vi "Argo_Drive.vi"(0 "Speed_Main":dbl=-0.047244094488188976, 1 "Turning_Still_Multiplier":dbl=1.5, 2 "Argo Drive Joystick Map":T1, 3 "Backwards_Turning_Flip":bool, 4 "Turning_PID_Enable":bool, 5 "PID Gains":T3, 6 "Turning_Main":dbl=-0.007874015748031496, 7 "Auto_Enable":bool, 8 "High_Gear":bool, 9 "Quick_Turn":bool=TRUE, 10 "Turning_Setpoint":dbl, 11 "dt (s)":dbl=10.0 format="%.3f", 14 "Yaw":dbl=654.9580428601698) -> (12 "Left_Motor":dbl format="%.2f", 13 "Right_Motor":dbl format="%.2f")   [LabVIEW 2017, in "ArgosLib.lvlib"]
uses:
  ArgosLib.lvlib
  Miscellaneous/TypeDefs/ArgoDriveJoystickMap.ctl
  Miscellaneous/TypeDefs/LookUpTableParameters.ctl
panel:
  out "Waveform Chart":cluster{"Left_Motor_Sat":dbl, "Output":dbl}(graph)
  in  "Ramp_Rate":dbl=0.2
  out "XY Turning":cluster{"Turning X ":dbl[], "Turning Y":dbl[]}(graph)={"Turning X "=[-1.0, -0.75, -0.2, -0.19, 0.0, 0.19, 0.2, 0.75, 1.0], "Turning Y"=[-1.0, -0.4, -0.1, 0.0, 0.0, 0.0, 0.1, 0.4, 1.0]}
  out "XY Speed":cluster{"Speed X":dbl[], "Speed Y":dbl[]}(graph)={"Speed X"=[-1.0, -0.75, -0.21, -0.2, 0.0, 0.2, 0.21, 0.75, 1.0], "Speed Y"=[-1.0, -0.4, -0.15, 0.0, 0.0, 0.0, 0.15, 0.4, 1.0]}
  in  "Turning Scale":dbl=1.5
  out "Delta":dbl format="%.2f"
  # "Chessy Drive"
  # "This subystem takes turning and speed controls from a xbox joystick \nand creats left and right motor values"
  # "Tunning"
  # "Inputs"
  # "Test Points"
  # "Ouputs"
  # "Joystick Map (Lookup Table)"
  # "Turning Power Mode"
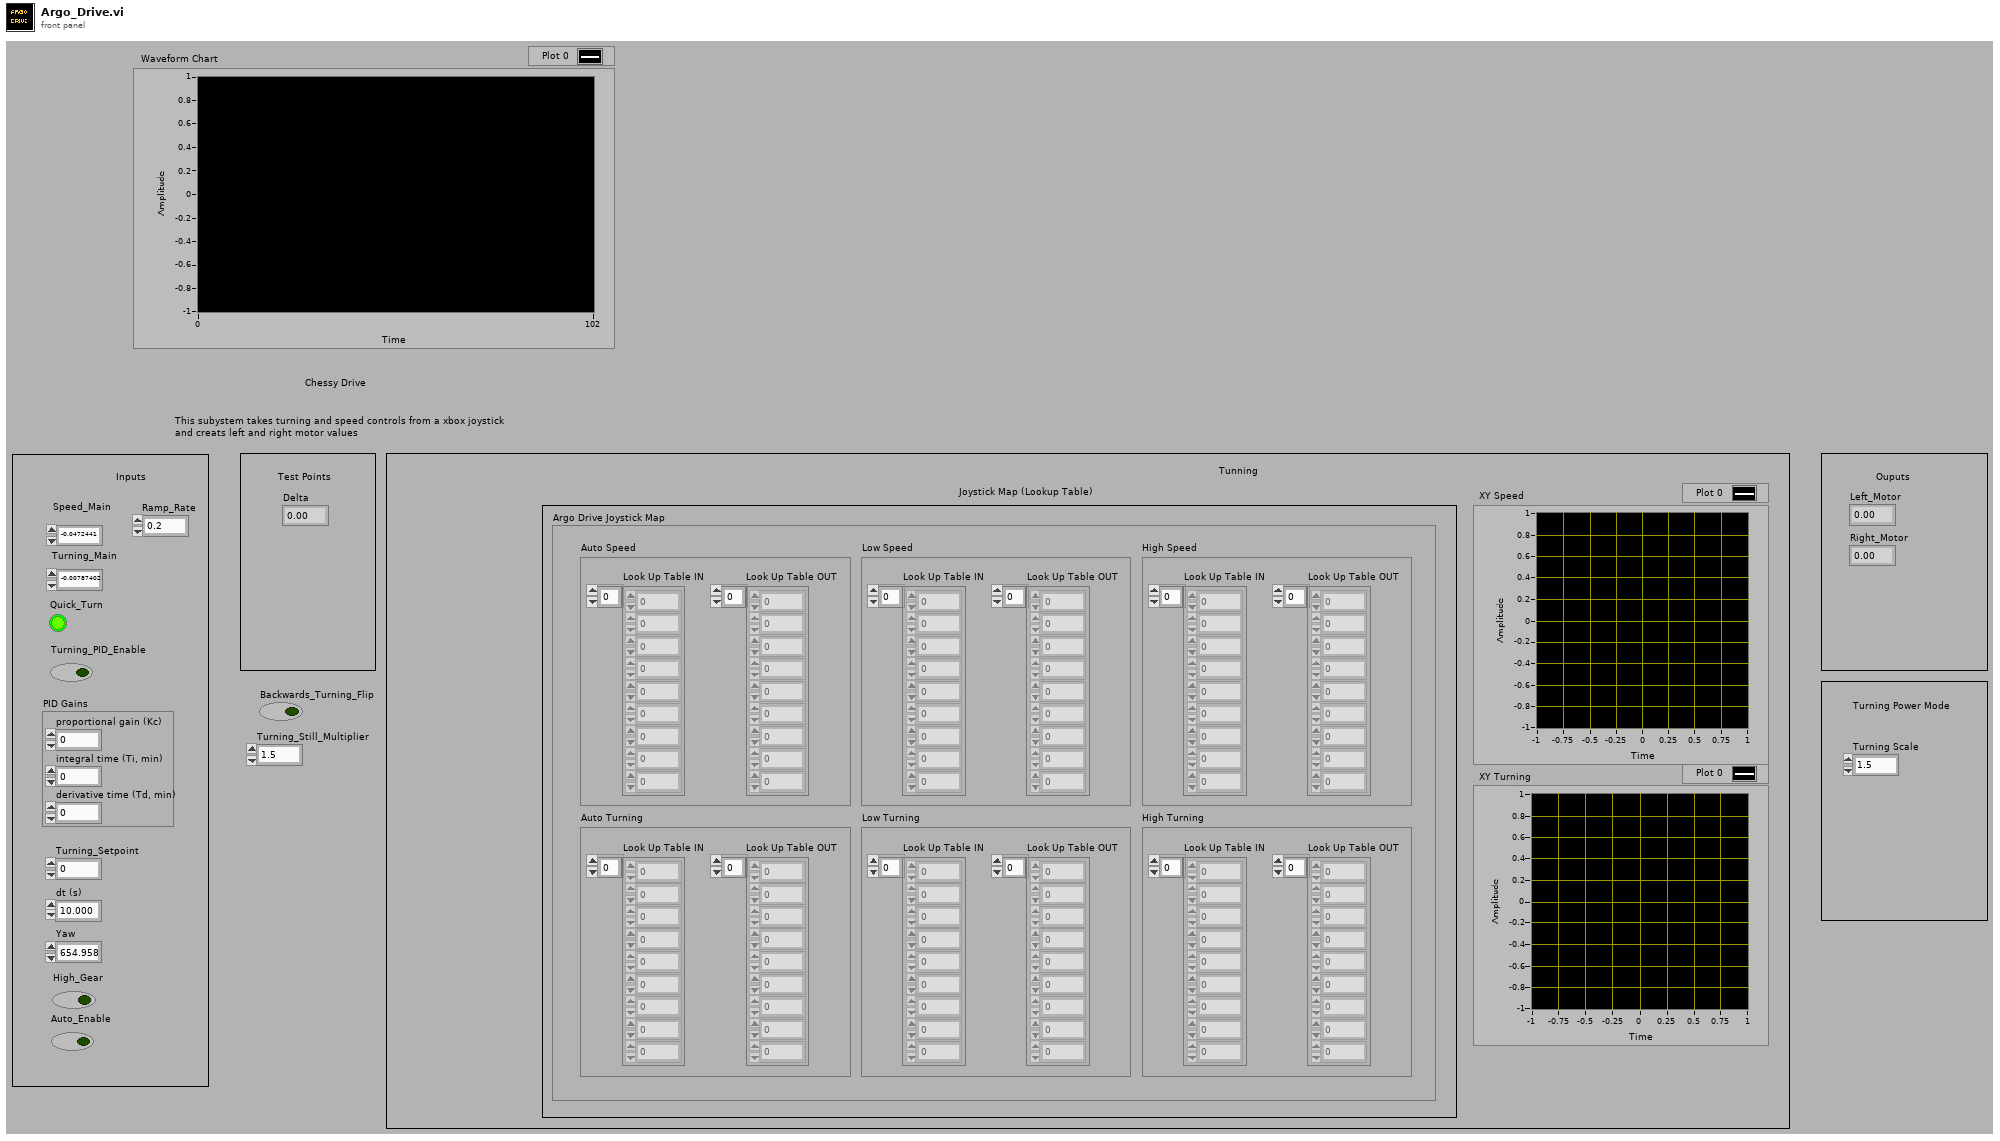
[diagram p1: front panel]
types:
  T1 = typedef "ArgosLib.lvlib/ArgoDriveJoystickMap.ctl" = cluster{"Auto Speed":T2, "Low Speed":T2, "Auto Turning":T2, "Low Turning":T2, "High Speed":T2, "High Turning":T2}
  T2 = typedef "ArgosLib.lvlib/LookUpTableParameters.ctl" = cluster{"Look Up Table OUT":dbl[], "Look Up Table IN":dbl[]}
  T3 = cluster{"proportional gain (Kc)":dbl, "integral time (Ti, min)":dbl, "derivative time (Td, min)":dbl}
  T4 = cluster{"Look Up Table IN":dbl[], "Look Up Table OUT":dbl[]}
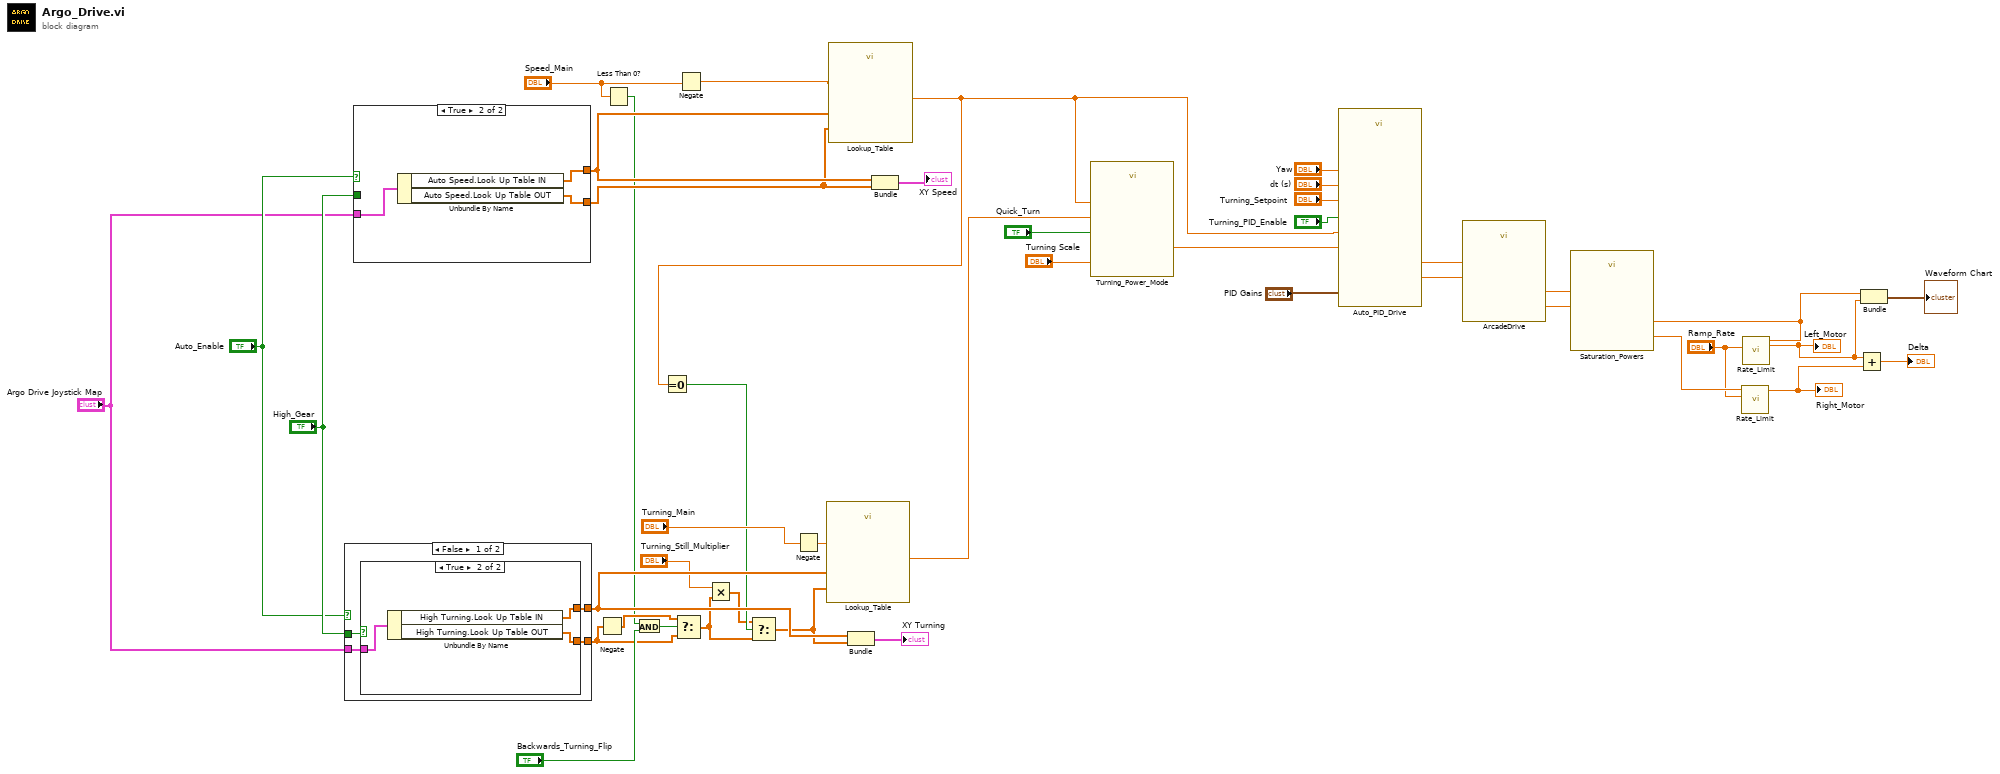
[diagram p0: block diagram]
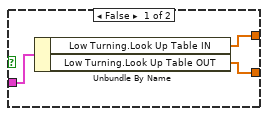
[diagram p2: hidden frame]
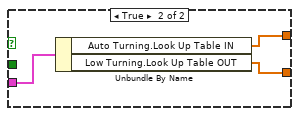
[diagram p3: hidden frame]
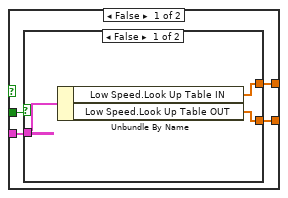
[diagram p4: hidden frame]
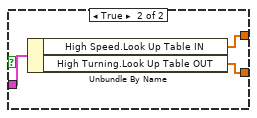
[diagram p5: hidden frame]
diagram:
  n1 = case shown="False" "Auto_Enable" {
    tunnel: "High_Gear" -> [w47 _]
    tunnel: [w46 w55] -> w27
    tunnel: [w45 w54] -> w10
    tunnel: "Argo Drive Joystick Map" -> [w44 w56]
    frame False {
      n2 = case shown="True" w47 {
        tunnel: [w49 w52] -> w46
        tunnel: [w48 w51] -> w45
        tunnel: w44 -> [w50 w53]
        frame False {
          n3 = Unbundle By Name(w50) -> ("Low Turning.Look Up Table IN"=w49:dbl[], "Low Turning.Look Up Table OUT"=w48:dbl[])
        }
        frame True {
          n4 = Unbundle By Name(w53) -> ("High Turning.Look Up Table IN"=w52:dbl[], "High Turning.Look Up Table OUT"=w51:dbl[])
        }
      }
    }
    frame True {
      n5 = Unbundle By Name(w56) -> ("Auto Turning.Look Up Table IN"=w55:dbl[], "Low Turning.Look Up Table OUT"=w54:dbl[])
    }
  }
  n6 = case shown="True" "Auto_Enable" {
    tunnel: "High_Gear" -> [w60 _]
    tunnel: [w59 w68] -> w29
    tunnel: [w58 w67] -> w28
    tunnel: "Argo Drive Joystick Map" -> [w57 w69]
    frame False {
      n7 = case shown="False" w60 {
        tunnel: [w62 w65] -> w59
        tunnel: [w61 w64] -> w58
        tunnel: w57 -> [w63 w66]
        frame False {
          n8 = Unbundle By Name(w63) -> ("Low Speed.Look Up Table IN"=w62:dbl[], "Low Speed.Look Up Table OUT"=w61:dbl[])
        }
        frame True {
          n9 = Unbundle By Name(w66) -> ("High Speed.Look Up Table IN"=w65:dbl[], "High Turning.Look Up Table OUT"=w64:dbl[])
        }
      }
    }
    frame True {
      n10 = Unbundle By Name(w69) -> ("Auto Speed.Look Up Table IN"=w68:dbl[], "Auto Speed.Look Up Table OUT"=w67:dbl[])
    }
  }
  n11 = Negate(x=w10) -> (-x=w9:dbl[])
  n12 = Less Than 0?(x="Speed_Main") -> (x < 0?=w7:bool)
  n13 = And(x=w7, y="Backwards_Turning_Flip") -> (x .and. y?=w11:bool)
  n14 = Select(t=w9, s=w11, f=w10) -> (s? t:f=w2:dbl[])
  n15 = Negate(x="Speed_Main") -> (-x=w22:dbl)
  n16 = Multiply(x="Turning_Still_Multiplier", y=w2) -> (x*y=w3:dbl[])
  n17 = Negate(x="Turning_Main") -> (-x=w25:dbl)
  n18 = call "Lookup_Table.vi"("Y_Array"=w28, "x_in"=w22, "X_Array"=w29) -> ("y_out"=w5:dbl)  [unwired: 6 in]
  n19 = Equal To 0?(x=w5) -> (x = 0?=w4:bool)
  n20 = Select(t=w3, s=w4, f=w2) -> (s? t:f=w6:dbl[])
  n21 = call "Lookup_Table.vi"("Y_Array"=w6, "x_in"=w25, "X_Array"=w27) -> ("y_out"=w37:dbl)  [unwired: 6 in]
  n22 = Bundle("Look Up Table IN"=w27, "Look Up Table OUT"=w6) -> (→"XY Turning":T4)  [unwired: 1 in]
  n23 = Bundle("Look Up Table IN"=w29, "Look Up Table OUT"=w28) -> (→"XY Speed":T4)  [unwired: 1 in]
  n24 = call "Turning_Power_Mode.vi"("Turning_Scale"="Turning Scale", "Quick_Turn"="Quick_Turn", "Turning"=w37, "Power"=w5) -> ("Turning_Correction"=w34:dbl)  [unwired: 7 in]
  n25 = call "Auto_PID_Drive.vi"("Power"=w5, "dt (s)"="dt (s)", "Turning"=w34, "PID Gains"="PID Gains", "Yaw"="Yaw", "Turning_Setpoint"="Turning_Setpoint", "Turning_PID_Enable"="Turning_PID_Enable") -> ("Power"=w36:dbl, "Turning"=w35:dbl)  [unwired: 7 in]
  n26 = call "ArcadeDrive.vi"("Turning"=w35, "Power"=w36) -> ("Right_Motor"=w42:dbl, "Left_Motor"=w41:dbl)  [unwired: 8 in]
  n27 = call "Saturation_Powers.vi"("Right_Motor"=w42, "Left_Motor"=w41) -> ("Right_Motor_Say"=w21:dbl, "Left_Motor_Sat"=w16:dbl)  [unwired: 8 in]
  n28 = call "Rate_Limit.vi"("Ramp_Rate"="Ramp_Rate", "Input"=w21) -> ("Output"=w19:dbl)  [unwired: 9 in]
  "Right_Motor" <- w19
  n29 = call "Rate_Limit.vi"("Ramp_Rate"="Ramp_Rate", "Input"=w16) -> ("Output"=w17:dbl)  [unwired: 9 in]
  "Left_Motor" <- w17
  n30 = Add(x=w17, y=w19) -> (x+y=→"Delta":dbl)
  n31 = Bundle("Left_Motor_Sat"=w16, "Output"=w17) -> (→"Waveform Chart":cluster{"Left_Motor_Sat":dbl, "Output":dbl})  [unwired: 1 in]
